vi "Perform Action.vi"(8 "error in (no error)":errorcluster, 10 "Input":variant, 11 "DIO DAQmx PWM Fixed Freq CFG in":refnum<class "DIO DAQmx PWM Fixed Freq CFG.lvclass">) -> (0 "error out":errorcluster, 2 "Output":variant, 3 "DIO DAQmx PWM Fixed Freq CFG out":refnum<class "DIO DAQmx PWM Fixed Freq CFG.lvclass">)   [LabVIEW 2023, in "DAQmx Simulated CFGs.lvlib" / "DIO DAQmx PWM Fixed Freq CFG.lvclass"]
uses:
  DIO DAQmx PWM Fixed Freq CFG.lvclass
  D:/git/HAL/HAL GOOP4/DAQmx/DAQmx Base CFG/DAQmx Base CFG.lvclass
  DAQmx/DAQmx Base CFG/DAQmx Base CFG.lvclass
panel:
  out "Duty Cycle":dbl
  out "resulting string":string
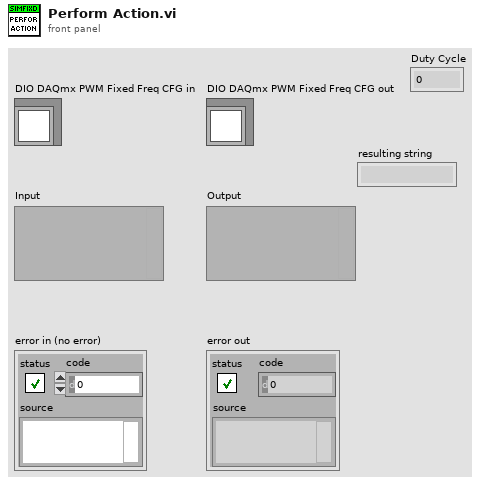
[diagram p1: front panel]
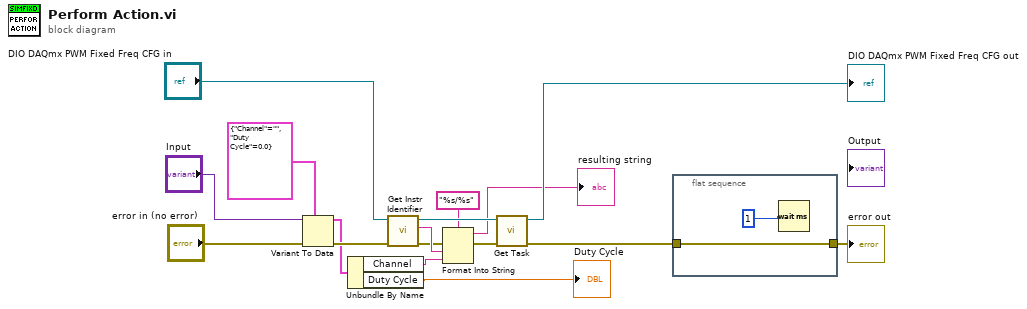
[diagram p0: block diagram]
diagram:
  n1 = Variant To Data(error in="error in (no error)", type=cluster{"Channel":string, "Duty Cycle":dbl} {"Channel"="", "Duty Cycle"=0.0}, Variant="Input") -> (data=w3:cluster{"Channel":string, "Duty Cycle":dbl}, error out=w17:errorcluster)
  n2 = Unbundle By Name(w3) -> ("Channel"=w2:string, "Duty Cycle"=→"Duty Cycle":dbl)
  n3 = call-dynamic "Get Instr Identifier.vi"("error in (no error)"=w17, "Configuration Base in"="DIO DAQmx PWM Fixed Freq CFG in") -> ("error out"=w13:errorcluster, "Instr Identifier"=w14:string, "Configuration Base out"=w16:refnum<class "DIO DAQmx PWM Fixed Freq CFG.lvclass">)  [unwired: 7 in]
  n4 = Format Into String(format string="%s/%s", error in=w13, w14, w2) -> (resulting string=→"resulting string":string, error out=w12:errorcluster)  [unwired: 1 in]
  n5 = call "Get Task.vi"("error in (no error)"=w12, "DAQmx Base CFG in"=w16) -> ("error out"=w6:errorcluster, "DAQmx Base CFG out"=→"DIO DAQmx PWM Fixed Freq CFG out":refnum<class "DIO DAQmx PWM Fixed Freq CFG.lvclass">)  [unwired: 7 in, 1 out]
  n6 = flat-sequence {
    tunnel: w6 -> [w19]
    tunnel: [w19] -> w5
    frame #0 {
      n7 = Wait (ms)(milliseconds to wait=u32 1) -> ()  [unwired: 1 out]
    }
  }
  "error out" <- w5
